vi "Retrieve roboRIO personality file.vi"(8 "error in (no error)":errorcluster, 10 "Message Queue":refnum<queue>, 11 "UI Data Out":T1) -> (0 "error out":errorcluster, 3 "UI Data in":T1)   [LabVIEW 2018, in "Personalities Tool.lvlib"]
doc: "This VI transfers a personality file from the roboRIO to the computer, then checks it against existing personalities locally and offers a diff, if needed."
uses:
  Personalities Tool.lvlib
  Controls/QMH Data.ctl
  Controls/Personality Type.ctl
  Controls/roboRIO Connection Information.ctl
  Message Queue/Message Cluster.ctl
  Message Queue/Enqueue Message (Single).vi
  <vilib>/FTP/NI_FTP.lvlib
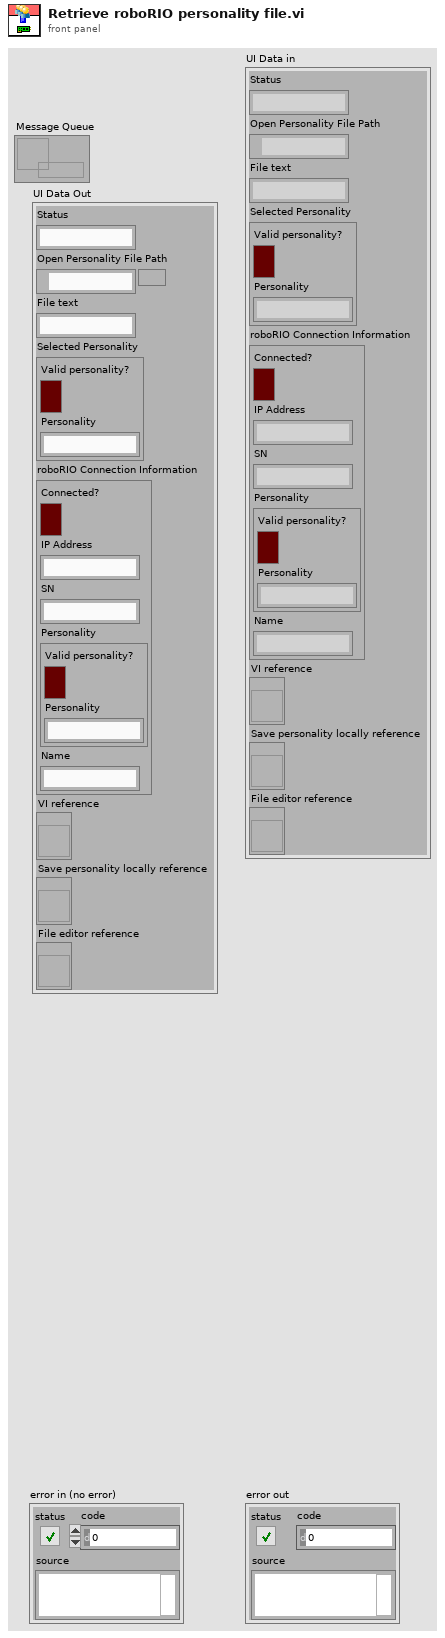
[diagram p1: front panel]
types:
  T1 = typedef "Personalities Tool.lvlib/QMH Data.ctl" = cluster{"Status":string, "Open Personality File Path":path, "File text":string, "Selected Personality":T2, "roboRIO Connection Information":T3, "VI reference":refnum<vi>, "Save personality locally reference":refnum<vi>, "File editor reference":refnum<vi>}
  T2 = typedef "Personalities Tool.lvlib/Personality Type.ctl" = cluster{"Valid personality?":bool, "Personality":string}
  T3 = typedef "Personalities Tool.lvlib/roboRIO Connection Information.ctl" = cluster{"Connected?":bool, "IP Address":string, "SN":string, "Personality":T2, "Name":string}
  T4 = typedef "Personalities Tool.lvlib/Diff Key.ctl" = cluster{"Section":string, "Local":variant, "roboRIO":variant, "Selection":enum32{"Item 0", "Item 1"}, "Key":string}
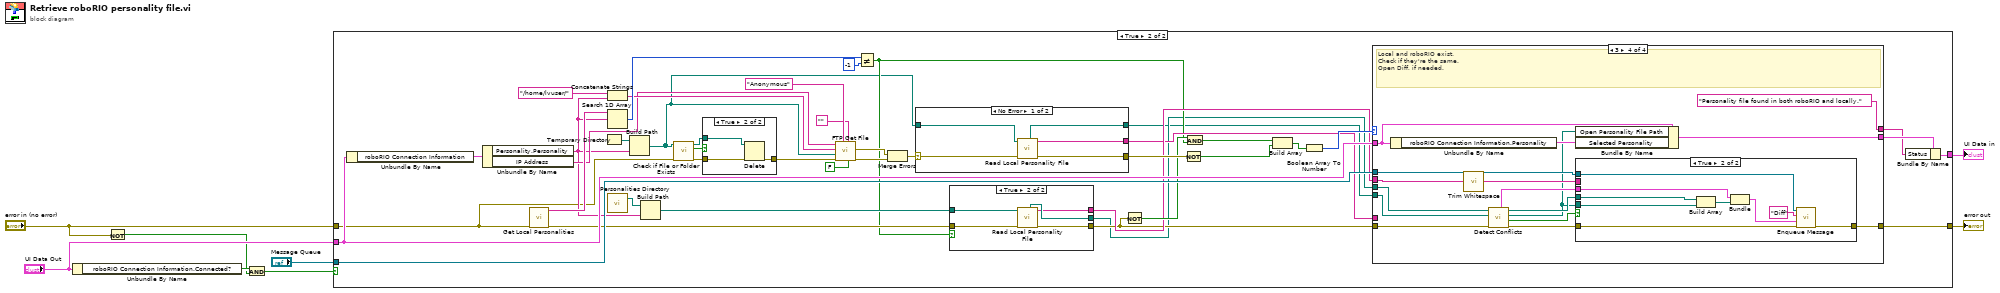
[diagram p0: block diagram]
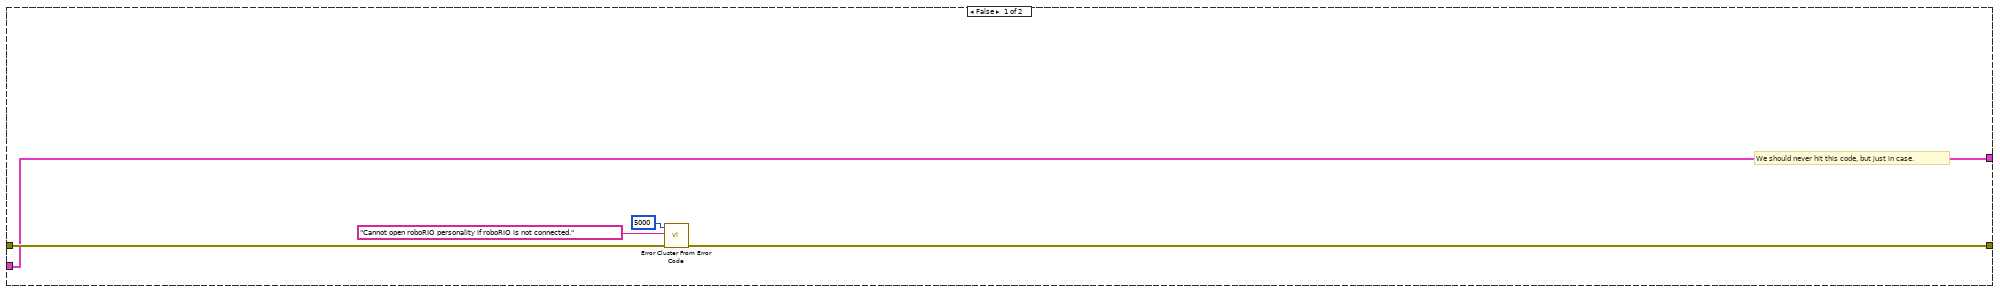
[diagram p2: hidden frame]
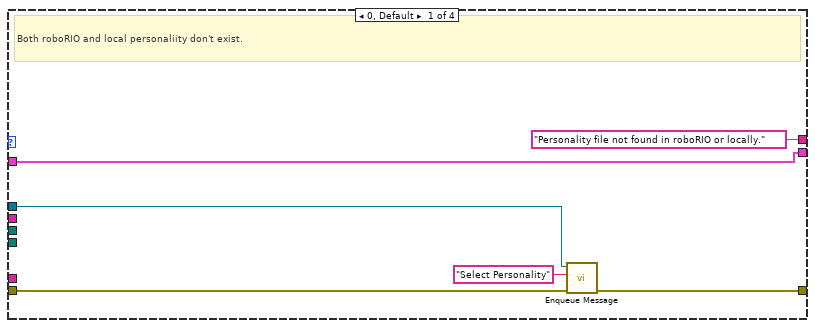
[diagram p6: hidden frame]
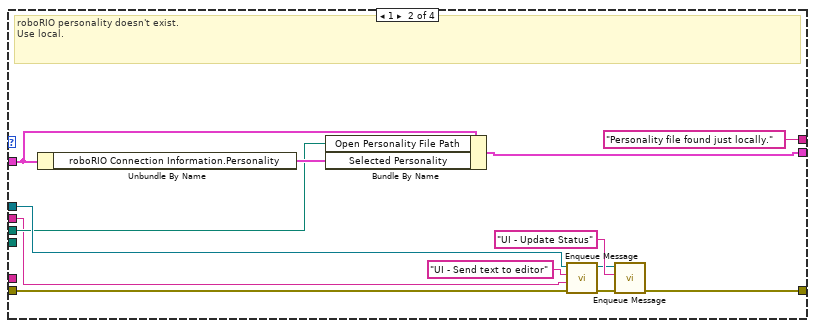
[diagram p7: hidden frame]
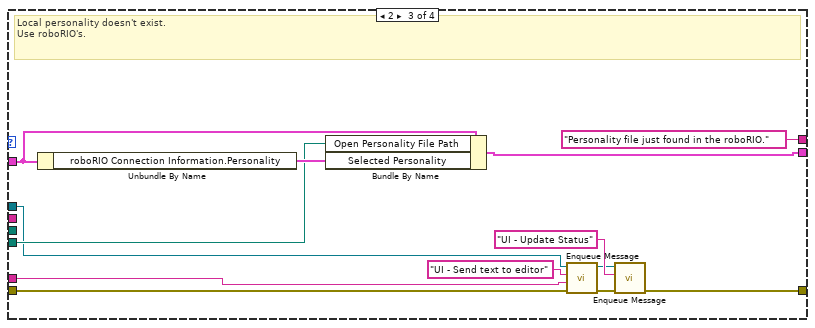
[diagram p8: hidden frame]
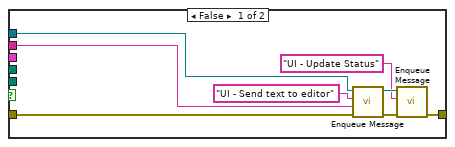
[diagram p9: hidden frame]
diagram:
  n1 = Unbundle By Name("UI Data Out") -> ("roboRIO Connection Information.Connected?"=w7:bool)
  n2 = Not(x="error in (no error)") -> (.not. x?=w3:bool)
  n3 = And(x=w7, y=w3) -> (x .and. y?=w4:bool)
  n4 = case shown="True" w4 {
    tunnel: [w12 w52] -> w5
    tunnel: "error in (no error)" -> [w13 w16]
    tunnel: "UI Data Out" -> [w11 w41]
    tunnel: [w11 w37] -> w6
    tunnel: "Message Queue" -> [_ w35]
    frame False {
      # "We should never hit this code, but just in case."
      n5 = call <vilib>:"Error Cluster From Error Code.vi"("error in (no error)"=w13, "error message (\"\")"="Cannot open roboRIO personality if roboRIO is not connected." ("error message (\"\")"), "error code (0)"=5000) -> ("error out"=w12:errorcluster)  [unwired: 6 in]
    }
    frame True {
      n6 = Unbundle By Name(w41) -> ("roboRIO Connection Information"=w42:T3)
      n7 = Unbundle By Name(w42) -> ("Personality.Personality"=w21:string, "IP Address"=w44:string)
      n8 = call "Get Local Personalities.vi"("error in (no error)"=w16) -> ("error out"=w31:errorcluster, "Personalities"=w53:string[])  [unwired: 9 in]
      n9 = Temporary Directory() -> (w45:path)
      n10 = Concatenate Strings("/home/lvuser/" ("string"), w21) -> (w49:string)
      n11 = Search 1D Array(1D array=w53, element=w21) -> (index of element=w55:i32)  [unwired: 1 in]
      n12 = call "Personalities Directory.vi"() -> ("appended path"=w34:path)  [unwired: 3 in]
      n13 = Build Path(base path=w45, name or relative path=w21) -> (appended path=w17:path)
      n14 = Build Path(base path=w34, name or relative path=w21) -> (appended path=w30:path)
      n15 = call <vilib>:"Check if File or Folder Exists.vi"("error in (no error)"=w16, "path"=w17) -> ("error out"=w19:errorcluster, "file or folder exists?"=w20:bool, "dup path"=w18:path)  [unwired: 7 in]
      n16 = case shown="True" w20 {
        tunnel: w19 -> [w56 w59]
        tunnel: w18 -> [_ w58]
        tunnel: [w56 w57] -> w15
        frame False {
        }
        frame True {
          n17 = Delete(path (use dialog)=w58, error in=w59) -> (error out=w57:errorcluster)  [unwired: 3 in, 2 out]
        }
      }
      n18 = call <vilib>:"FTP Get File.vi"("active (T)"=FALSE, "password"="", "user"="Anonymous" ("username"), "error in (no error)"=w15, "local path"=w17, "remote path"=w49, "host"=w44) -> ("error out"=w48:errorcluster, "file error"=w47:errorcluster)  [unwired: 3 in]
      n19 = Not Equal?(x=w55, y=-1) -> (x != y?=w26:bool)
      n20 = Merge Errors(w47, w48) -> (w33:errorcluster)
      n21 = case shown="No Error" w33 {
        selector: w33 -> [w71 w73]
        tunnel: [w70 w73] -> w32
        tunnel: w17 -> [w69 w72]
        tunnel: [w68 w72] -> w22
        tunnel: [w67 _] -> w27
        frame No Error {
          n22 = call "Read Local Personality File.vi"("error in (no error)"=w71, "File Path"=w69) -> ("error out"=w70:errorcluster, "Personality text"=w67:string, "path"=w68:path)  [unwired: 7 in]
        }
        frame Error {
        }
      }
      n23 = case shown="True" w26 {
        tunnel: w31 -> [w61 w66]
        tunnel: [w61 w65] -> w25
        tunnel: w30 -> [w60 w64]
        tunnel: [w60 w63] -> w23
        tunnel: [_ w62] -> w28
        frame False {
        }
        frame True {
          n24 = call "Read Local Personality File.vi"("error in (no error)"=w66, "File Path"=w64) -> ("error out"=w65:errorcluster, "Personality text"=w62:string, "path"=w63:path)  [unwired: 7 in]
        }
      }
      n25 = Not(x=w25) -> (.not. x?=w29:bool)
      n26 = Not(x=w32) -> (.not. x?=w40:bool)
      n27 = And(x=w29, y=w26) -> (x .and. y?=w24:bool)
      n28 = Build Array(w24, w40) -> (w39:bool[])
      n29 = Boolean Array To Number(Boolean array=w39) -> (number=w38:u32)
      n30 = case shown="3" w38 {
        tunnel: w25 -> [w79 w83 w96 w115]
        tunnel: [w76 w81 w97 w120] -> w52
        tunnel: w41 -> [w78 w90 w103 w117]
        tunnel: [w78 w91 w102 w107] -> w43
        tunnel: ["Personality file not found in roboRIO or locally." ("Status") "Personality file found just locally." ("Status") "Personality file just found in the roboRIO." ("Status") "Personality file found in both roboRIO and locally." ("Status")] -> w36
        tunnel: w35 -> [w75 w84 w94 w119]
        tunnel: w22 -> [_ _ w95 w113]
        tunnel: w23 -> [_ w82 _ w114]
        tunnel: w28 -> [_ w80 _ w118]
        tunnel: w27 -> [_ _ w93 _]
        frame 0, Default {
          # "Both roboRIO and local personaliity don't exist."
          n31 = call-poly "Enqueue Message.vi"("error in (no error)"=w79, "Message"="Select Personality", "Message Queue"=w75) -> ("error out"=w76:errorcluster)  [unwired: 7 in, 1 out]
        }
        frame 1 {
          # "roboRIO personality doesn't exist.\nUse local."
          n32 = Unbundle By Name(w90) -> ("roboRIO Connection Information.Personality"=w89:T2)
          n33 = Bundle By Name(cluster=w90, "Open Personality File Path"=w82, "Selected Personality"=w89) -> (w91:T1)
          n34 = call-poly "Enqueue Message.vi"("error in (no error)"=w83, "Message Data"=w80, "Message"="UI - Send text to editor", "Message Queue"=w84) -> ("error out"=w85:errorcluster, "dup Message Queue"=w86:refnum<queue>)  [unwired: 6 in]
          n35 = call-poly "Enqueue Message.vi"("error in (no error)"=w85, "Message"="UI - Update Status", "Message Queue"=w86) -> ("error out"=w81:errorcluster)  [unwired: 7 in, 1 out]
        }
        frame 2 {
          # "Local personality doesn't exist. \nUse roboRIO's."
          n36 = Unbundle By Name(w103) -> ("roboRIO Connection Information.Personality"=w104:T2)
          n37 = Bundle By Name(cluster=w103, "Open Personality File Path"=w95, "Selected Personality"=w104) -> (w102:T1)
          n38 = call-poly "Enqueue Message.vi"("error in (no error)"=w96, "Message Data"=w93, "Message"="UI - Send text to editor", "Message Queue"=w94) -> ("error out"=w98:errorcluster, "dup Message Queue"=w99:refnum<queue>)  [unwired: 6 in]
          n39 = call-poly "Enqueue Message.vi"("error in (no error)"=w98, "Message"="UI - Update Status", "Message Queue"=w99) -> ("error out"=w97:errorcluster)  [unwired: 7 in, 1 out]
        }
        frame 3 {
          # "Local and roboRIO exist.\nCheck if they're the same.\nOpen Diff, if needed."
          n40 = Unbundle By Name(w117) -> ("roboRIO Connection Information.Personality"=w108:T2)
          n41 = call <vilib>:"Trim Whitespace.vi"("string"=w118) -> ("trimmed string"=w116:string)  [unwired: 1 in]
          n42 = call "Detect Conflicts.vi"("error in (no error)"=w115, "roboRIO"=w113, "Local"=w114) -> ("error out"=w112:errorcluster, "Conflicts?"=w110:bool, "roboRIO out"=w106:path, "Local out"=w109:path, "Items with conflicts"=w111:T4[])  [unwired: 4 in]
          n43 = Bundle By Name(cluster=w117, "Open Personality File Path"=w106, "Selected Personality"=w108) -> (w107:T1)
          n44 = case shown="True" w110 {
            tunnel: w112 -> [w124 w138]
            tunnel: [w125 w137] -> w120
            tunnel: w119 -> [w123 w136]
            tunnel: w109 -> [_ w134]
            tunnel: w106 -> [_ w133]
            tunnel: w116 -> [w122 _]
            tunnel: w111 -> [_ w130]
            frame False {
              n45 = call-poly "Enqueue Message.vi"("error in (no error)"=w124, "Message Data"=w122, "Message"="UI - Send text to editor", "Message Queue"=w123) -> ("error out"=w129:errorcluster, "dup Message Queue"=w128:refnum<queue>)  [unwired: 6 in]
              n46 = call-poly "Enqueue Message.vi"("error in (no error)"=w129, "Message"="UI - Update Status", "Message Queue"=w128) -> ("error out"=w125:errorcluster)  [unwired: 7 in, 1 out]
            }
            frame True {
              n47 = Build Array(w134, w133) -> (w132:path[])
              n48 = Bundle("Items with conflicts"=w130, w132) -> (w131:cluster{"Items with conflicts":T4[], path[]})  [unwired: 1 in]
              n49 = call-poly "Enqueue Message.vi"("error in (no error)"=w138, "Message Data"=w131, "Message"="Diff", "Message Queue"=w136) -> ("error out"=w137:errorcluster)  [unwired: 6 in, 1 out]
            }
          }
        }
      }
      n50 = Bundle By Name(cluster=w43, "Status"=w36) -> (w37:T1)
    }
  }
  "UI Data in" <- w6
  "error out" <- w5
